vi "TCP Daemon.vi"(8 "UUID":string, 9 "Super Data Model":refnum<class "Super Data Model.lvclass">, 10 "transmission data unit":refnum<class "Transmission Data Unit.lvclass">, 11 "TCP slave in":refnum<class "TCP Slave.lvclass">) -> ()   [LabVIEW 2013, in "Modbus Library - Advance.lvlib" / "TCP Slave.lvclass"]
doc: "This daemon waits for new connections and launches connection handlers as needed. It also obtains a local reference to the quit notification, and waits for that to occur."
uses:
  TCP Slave.lvclass
  Transmission Data Unit/Transmission Data Unit.lvclass
  Super Data Model/Super Data Model.lvclass
  Listener State.ctl
  daemon status.ctl
  Network Slave.lvclass/Network Slave.ctl
  TCP Slave.lvclass/TCP Slave.ctl
  Remove Unused Connections.vi
  Network Slave.lvclass
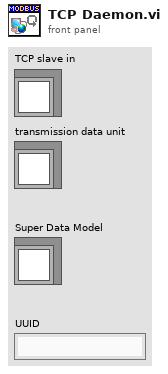
[diagram p1: front panel]
types:
  T1 = typedef "Modbus Library - Advance.lvlib/TCP Slave.lvclass/Listener State.ctl" = enum16{"Check Notifier", "Check for Available Connection Slot", "Wait on Connection", "Quit"}
  T2 = typedef "Modbus Library - Advance.lvlib/Network Slave.lvclass/daemon status.ctl" = enum16{"Not Started", "Running", "Error", "Stopped"}
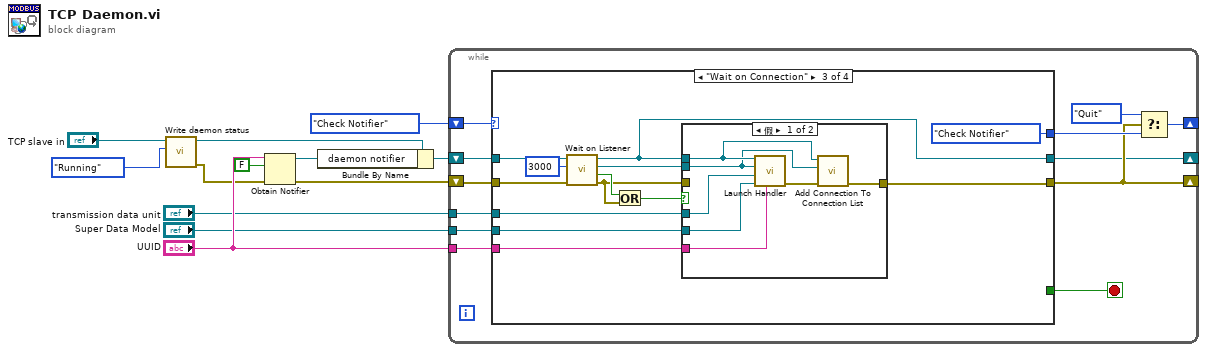
[diagram p0: block diagram]
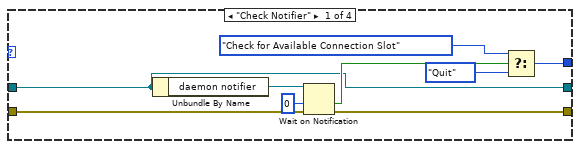
[diagram p2: hidden frame]
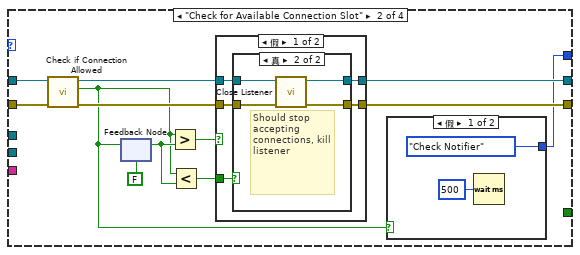
[diagram p3: hidden frame]
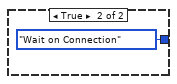
[diagram p4: hidden frame]
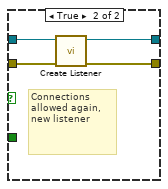
[diagram p6: hidden frame]
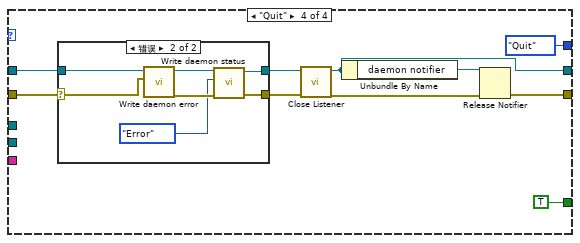
[diagram p8: hidden frame]
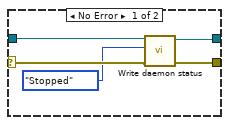
[diagram p9: hidden frame]
diagram:
  n1 = call "Write daemon status.vi"("daemon status"=daemon_status."Running", "Network Slave in"="TCP slave in") -> ("error out"=w2:errorcluster, "Network Slave out"=w4:refnum<class "TCP Slave.lvclass">)  [unwired: 8 in]
  n2 = Obtain Notifier(name (unnamed)="UUID", notification data type=FALSE, error in (no error)=w2) -> (notifier out=w10:refnum<notifier>, error out=w5:errorcluster)  [unwired: 1 in, 1 out]
  n3 = Bundle By Name(cluster=w4, "daemon notifier"=w10) -> (w9:refnum<class "TCP Slave.lvclass">)
  n4 = while {
    shift-right: [w22] -> _
    shift-left: Listener_State."Check Notifier" -> [w24]
    tunnel: "UUID" -> [w19]
    tunnel: "Super Data Model" -> [w18]
    tunnel: "transmission data unit" -> [w17]
    shift-right: [w16] -> _
    shift-left: w5 -> [w15]
    shift-right: [w13] -> _
    shift-left: w9 -> [w23]
    stop <- w14 stop-if-true
    n5 = case shown="\"Wait on Connection\"" w24 {
      tunnel: w23 -> [w25 w44 w75 w93]
      tunnel: [w32 w38 w65 w90] -> w16
      tunnel: [w27 w34 Listener_State."Check Notifier" Listener_State."Quit"] -> w20
      tunnel: w19 -> [_ _ w70 _]
      tunnel: w18 -> [_ _ w69 _]
      tunnel: w17 -> [_ _ w68 _]
      tunnel: w15 -> [w26 w45 w67 w94]
      tunnel: [_ _ _ TRUE] -> w14
      tunnel: [w25 w39 w66 w85] -> w13
      frame "Check Notifier" {
        n6 = Unbundle By Name(w25) -> ("daemon notifier"=w33:refnum<notifier>)
        n7 = Wait on Notification(notifier=w33, timeout in ms (-1)=0, error in (no error)=w26) -> (timed out?=w31:bool, error out=w32:errorcluster)  [unwired: 1 in, 2 out]
        n8 = Select(t=Listener_State."Check for Available Connection Slot", s=w31, f=Listener_State."Quit") -> (s? t:f=w27:T1)
      }
      frame "Check for Available Connection Slot" {
        n9 = call "Check if Connection Allowed.vi"("error in (no error)"=w45, "TCP Slave in"=w44) -> ("error out"=w41:errorcluster, "Connection Allowed"=w35:bool, "TCP Slave out"=w40:refnum<class "TCP Slave.lvclass">)  [unwired: 7 in]
        n10 = feedback-in #1(w35) -> ()
        n11 = feedback #1(FALSE) -> (w37:bool)
        n12 = Greater?(x=w35, y=w37) -> (0:w42:bool)
        n13 = Less?(x=w35, y=w37) -> (x < y?=w36:bool)
        n14 = case shown="假" w42 {
          tunnel: w41 -> [w51 w62]
          tunnel: w40 -> [w52 w63]
          tunnel: [w49 w61] -> w39
          tunnel: [w50 w60] -> w38
          tunnel: w36 -> [w53 _]
          frame False {
            n15 = case shown="真" w53 {
              tunnel: w52 -> [w55 w59]
              tunnel: w51 -> [w54 w58]
              tunnel: [w54 w57] -> w50
              tunnel: [w55 w56] -> w49
              frame False {
              }
              frame True {
                # "Should stop accepting connections, kill listener"
                n16 = call "Close Listener.vi"("error in"=w58, "TCP slave in"=w59) -> ("error out"=w57:errorcluster, "TCP slave out"=w56:refnum<class "TCP Slave.lvclass">)  [unwired: 8 in]
              }
            }
          }
          frame True {
            # "Connections allowed again, new listener"
            n17 = call "Create Listener.vi"("error in"=w62, "TCP slave in"=w63) -> ("error out"=w60:errorcluster, "TCP slave out"=w61:refnum<class "TCP Slave.lvclass">)  [unwired: 8 in]
          }
        }
        n18 = case shown="假" w35 {
          tunnel: [Listener_State."Check Notifier" Listener_State."Wait on Connection"] -> w34
          frame False {
            n19 = Wait (ms)(milliseconds to wait=u32 500) -> ()  [unwired: 1 out]
          }
          frame True {
          }
        }
      }
      frame "Wait on Connection" {
        n20 = call-dynamic "Wait on Listener.vi"("error in"=w67, "timeout ms (wait forever: -1)"=3000, "TCP slave in"=w75) -> ("error out"=w64:errorcluster, "Timed Out"=w73:bool, "connection reference"=w71:refnum<data-value>, "TCP slave out"=w66:refnum<class "TCP Slave.lvclass">)  [unwired: 5 in]
        n21 = Or(x=w73, y=w64) -> (x .or. y?=w72:bool)
        n22 = case shown="假" w72 {
          tunnel: w71 -> [w77 _]
          tunnel: w66 -> [w78 _]
          tunnel: w70 -> [w83 _]
          tunnel: w69 -> [w82 _]
          tunnel: w68 -> [w81 _]
          tunnel: [w80 w84] -> w65
          tunnel: w64 -> [_ w84]
          frame False {
            n23 = call "Launch Handler.vi"("UUID"=w83, "Super Data Model"=w82, "transmission data unit"=w81, "connection reference"=w77, "TCP slave"=w78) -> ("error out"=w79:errorcluster)  [unwired: 6 in]
            n24 = call "Add Connection To Connection List.vi"("error in"=w79, "data value reference"=w77, "TCP Slave in"=w78) -> ("error out"=w80:errorcluster)  [unwired: 8 in]
          }
          frame True {
          }
        }
      }
      frame "Quit" {
        n25 = case shown="错误" w94 {
          selector: w94 -> [w96 w101]
          tunnel: [w97 w103] -> w92
          tunnel: w93 -> [w99 w106]
          tunnel: [w98 w104] -> w91
          frame No Error {
            n26 = call "Write daemon status.vi"("error in (no error)"=w96, "daemon status"=daemon_status."Stopped", "Network Slave in"=w99) -> ("error out"=w97:errorcluster, "Network Slave out"=w98:refnum<class "TCP Slave.lvclass">)  [unwired: 7 in]
          }
          frame Error {
            n27 = call "Write daemon error.vi"("daemon error"=w101, "Network Slave in"=w106) -> ("error out"=w102:errorcluster, "Network Slave out"=w105:refnum<class "TCP Slave.lvclass">)  [unwired: 8 in]
            n28 = call "Write daemon status.vi"("error in (no error)"=w102, "daemon status"=daemon_status."Error", "Network Slave in"=w105) -> ("error out"=w103:errorcluster, "Network Slave out"=w104:refnum<class "TCP Slave.lvclass">)  [unwired: 7 in]
          }
        }
        n29 = call "Close Listener.vi"("error in"=w92, "TCP slave in"=w91) -> ("error out"=w86:errorcluster, "TCP slave out"=w85:refnum<class "TCP Slave.lvclass">)  [unwired: 8 in]
        n30 = Unbundle By Name(w85) -> ("daemon notifier"=w87:refnum<notifier>)
        n31 = Release Notifier(notifier=w87, error in (no error)=w86) -> (error out=w90:errorcluster)  [unwired: 1 in, 2 out]
      }
    }
    n32 = Select(t=Listener_State."Quit", s=w16, f=w20) -> (s? t:f=w22:T1)
  }
